vi "Read Log Content.vi"(8 "error in (no error)":errorcluster, 11 "Debug Log In":refnum<class "Debug Log.lvclass">) -> (0 "error out":errorcluster, 2 "Data Log":refnum<class "Debug Data.lvclass">[](array[class]), 3 "Debug Log Out":refnum<class "Debug Log.lvclass">)   [LabVIEW 2020, in "Debug Log.lvclass"]
uses:
  Debug Log.lvclass
  Debug Data/Debug Data.lvclass
  Debug Log.lvclass/Debug Log.ctl
  Filter/Filter.lvclass
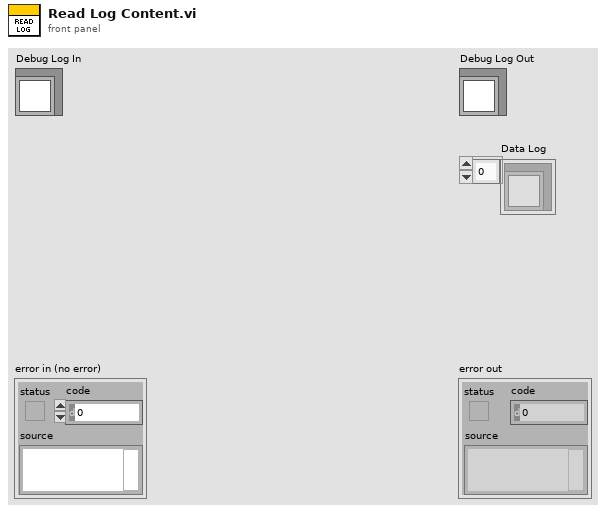
[diagram p1: front panel]
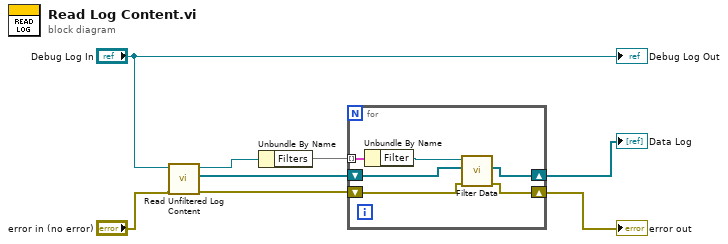
[diagram p0: block diagram]
diagram:
  n1 = call "Read Unfiltered Log Content.vi"("error in (no error)"="error in (no error)", "Debug Log In"="Debug Log In") -> ("error out"=w3:errorcluster, "Data Log"=w1:refnum<class "Debug Data.lvclass">[], "Debug Log Out"=w2:refnum<class "Debug Log.lvclass">)  [unwired: 7 in]
  n2 = Unbundle By Name(w2) -> ("Filters"=w8:map{string, refnum<class "Filter.lvclass">})
  n3 = for {
    tunnel: w8 -> [w14] mode=indexing
    shift-right: [w11] -> w7
    shift-left: w1 -> [w12]
    shift-right: [w9] -> w6
    shift-left: w3 -> [w10]
    n4 = Unbundle By Name(w14) -> ("Filter"=w13:refnum<class "Filter.lvclass">)
    n5 = call-dynamic "Filter Data.vi"("error in (no error)"=w10, "Debug Data In"=w12, "Filter in"=w13) -> ("error out"=w9:errorcluster, "Debug Data Out"=w11:refnum<class "Debug Data.lvclass">[])  [unwired: 6 in, 1 out]
  }
  "error out" <- w6
  "Data Log" <- w7
  "Debug Log Out" <- "Debug Log In"
